vi "Read Ch Names dyn.vi"(8 "error in (no error)":errorcluster, 11 "MKS in":refnum<class "MKS.lvclass">) -> (0 "error out":errorcluster, 2 "Ch Names":string[](array[string]), 3 "MKS out":refnum<class "MKS.lvclass">)   [LabVIEW 2022 SP3, in "MKS.lvclass"]
uses:
  MKS.lvclass
  MKS.lvclass/MKS.ctl
  hk-channel-class/hk-channel-class/HK Item/HK Item.lvclass
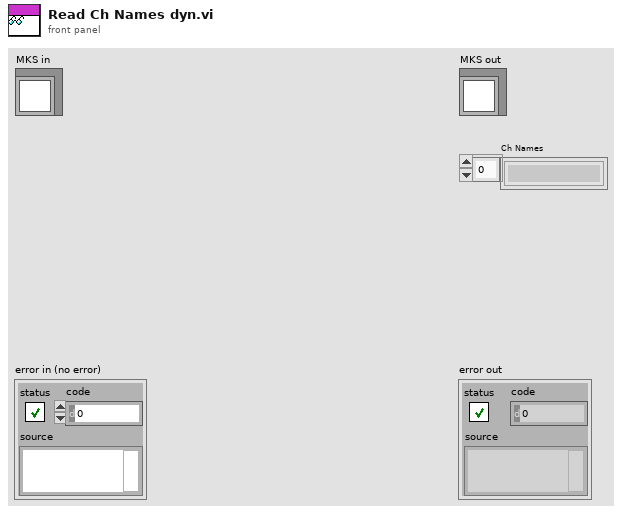
[diagram p1: front panel]
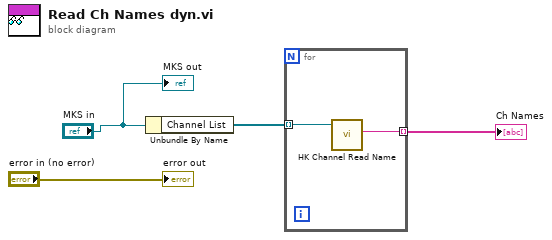
[diagram p0: block diagram]
diagram:
  n1 = Unbundle By Name("MKS in") -> ("Channel List"=w4:refnum<class "HK Item.lvclass">[])
  n2 = for {
    tunnel: w4 -> [w6] mode=indexing
    tunnel: [w5] -> w3 mode=indexing
    n3 = call "HK Channel Read Name.vi"("HK Item in"=w6) -> ("Name"=w5:string)  [unwired: 8 in, 2 out]
  }
  "Ch Names" <- w3
  "error out" <- "error in (no error)"
  "MKS out" <- "MKS in"
